vi "Handle Error (User).vi"(8 "error in":errorcluster, 11 "Node in":refnum<class "BLS Climate Chamber Template.lvclass">=refnum) -> (0 "error out":errorcluster, 3 "Node out":refnum<class "BLS Climate Chamber Template.lvclass">)   [LabVIEW 2023, in "BLS Climate Chamber Template.lvlib" / "BLS Climate Chamber Template.lvclass"]
uses:
  BLS Climate Chamber Template.lvclass
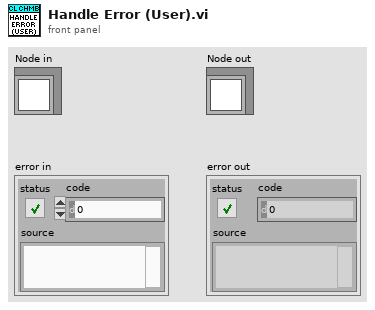
[diagram p1: front panel]
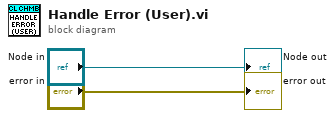
[diagram p0: block diagram]
diagram:
  "error out" <- "error in"
  "Node out" <- "Node in"
